vi "SUB sub_spectrogram.vi"(1 "scale info":variant, 2 "Bandwidth":cluster{"frequency":dbl, "+- f":dbl}={"frequency"=444.0, "+- f"=50.0}, 3 "scalogram matrix":cdb[][](array[numeric])) -> (0 "sub_Spectrogram":cdb[][](array[numeric]))   [LabVIEW 2017]
uses:
  <vilib>/addons/_Advanced Signal Processing/NI_AdvSigProcWA.lvlib
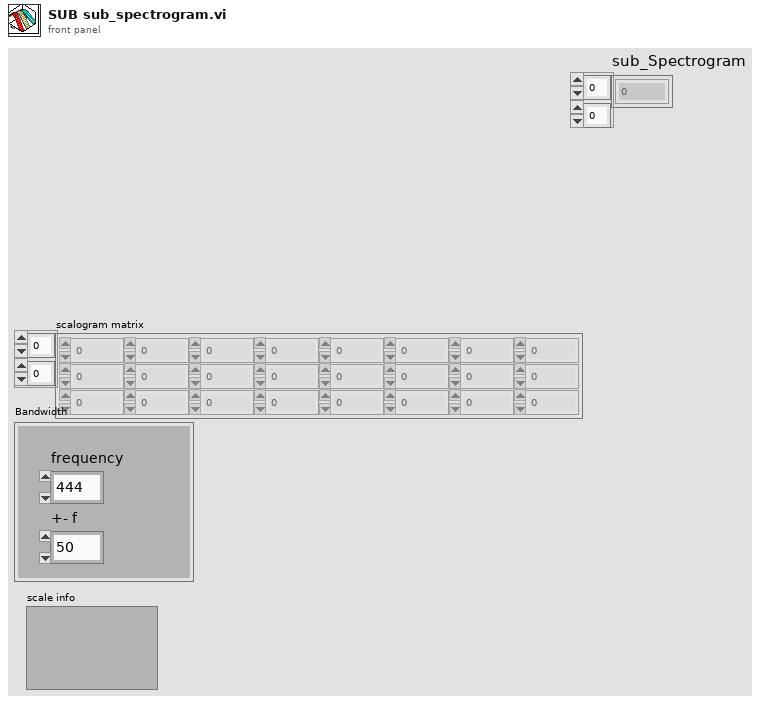
[diagram p1: front panel]
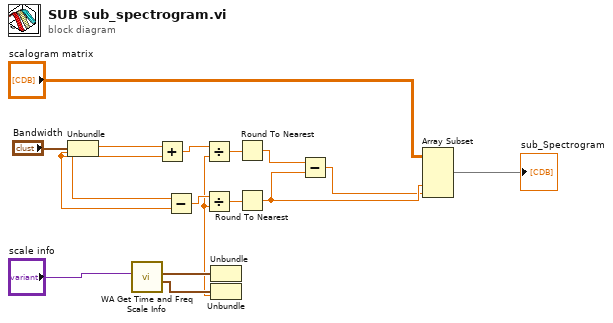
[diagram p0: block diagram]
diagram:
  n1 = Unbundle("Bandwidth") -> ("frequency"=w9:dbl, "+- f"=w8:dbl)
  n2 = call <vilib>:"WA Get Time and Freq Scale Info.vi"("scale info"="scale info") -> ("frequency info"=w16:cluster{"offset":dbl, "multiplier":dbl}, "time info"=w15:cluster{"offset":dbl, "multiplier":dbl})  [unwired: 1 in, 8 out]
  n3 = Add(x=w9, y=w8) -> (x+y=w7:dbl)
  n4 = Subtract(x=w9, y=w8) -> (x-y=w13:dbl)
  n5 = Unbundle(w15) -> ()  [unwired: 2 out]
  n6 = Unbundle(w16) -> ("multiplier"=w5:dbl)  [unwired: 1 out]
  n7 = Divide(x=w7, y=w5) -> (x/y=w6:dbl)
  n8 = Divide(x=w13, y=w5) -> (x/y=w12:dbl)
  n9 = Round To Nearest(number=w6) -> (nearest integer value=w4:dbl)
  n10 = Round To Nearest(number=w12) -> (nearest integer value=w3:dbl)
  n11 = Subtract(x=w4, y=w3) -> (x-y=w2:dbl)
  n12 = Array Subset(array="scalogram matrix", index (col)=w3, length (col)=w2) -> (→"sub_Spectrogram":cdb[][])  [unwired: 2 in]
